vi "M02 Toy Factory.vi"(9 "Angle in":dbl format="%#_13g", 11 "EV3 in":T1) -> (3 "EV3 out":T1)   [LabVIEW 2016]
uses:
  <vilib>/NXT/Subs/LVHSConnector.ctl
  <vilib>/NXT/LegoClasses/BrickReference/BrickReference.lvclass
  <vilib>/NXT/Dual Mode Library/Waits/Wait_Num.vi
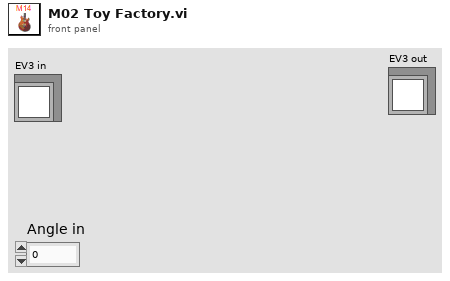
[diagram p1: front panel]
types:
  T1 = typedef "LVHSConnector.ctl" = refnum<class "BrickReference.lvclass">
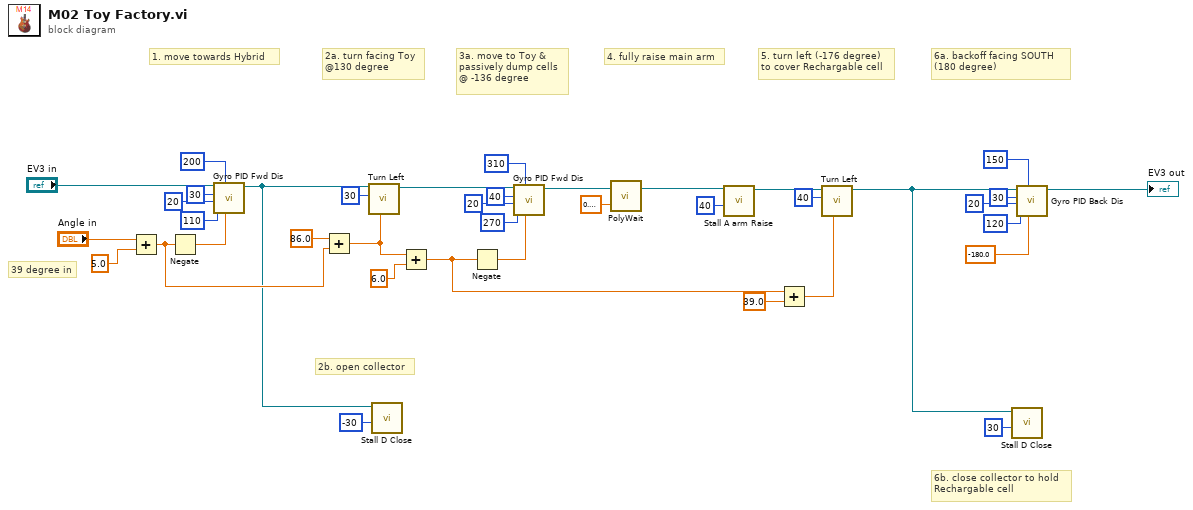
[diagram p0: block diagram]
diagram:
  # "39 degree in"
  # "6b. close collector to hold\nRechargable cell"
  # "2b. open collector"
  # "6a. backoff facing SOUTH\n(180 degree)"
  # "5. turn left (-176 degree)\nto cover Rechargable cell"
  # "4. fully raise main arm"
  # "3a. move to Toy &\npassively dump cells\n@ -136 degree"
  # "2a. turn facing Toy\n@130 degree"
  # "1. move towards Hybrid"
  n1 = Add(x="Angle in", y=5.0) -> (x+y=w30:dbl)
  n2 = Negate(x=w30) -> (-x=w28:dbl)
  n3 = call "Gyro PID Fwd Dis.vi"("Target angle"=w28, "Threshold to stop"=200 ("Stop rotation"), "Threshold to slow"=110 ("Threshold to De-acc"), "Min. speed"=20 ("De-acc"), "Max. speed"=30 ("Acc"), "EV3 in"="EV3 in") -> ("EV3 out"=w10:T1)  [unwired: 5 in]
  n4 = Add(x=86.0, y=w30) -> (x+y=w36:dbl)
  n5 = call "Turn Left.vi"("Turning angle"=w36, "Motor B (right)"=i8 30, "EV3 in"=w10) -> ("EV3 out"=w6:T1)  [unwired: 8 in]
  n6 = call "Stall D Close.vi"("Power"=i8 -30, "NXT/EV3"=w10) -> ()  [unwired: 9 in, 1 out]
  n7 = Add(x=w36, y=6.0) -> (x+y=w16:dbl)
  n8 = Negate(x=w16) -> (-x=w2:dbl)
  n9 = call "Gyro PID Fwd Dis.vi"("Target angle"=w2, "Threshold to stop"=310 ("Stop rotation"), "Threshold to slow"=270 ("Threshold to De-acc"), "Min. speed"=20 ("De-acc"), "Max. speed"=40 ("Acc"), "EV3 in"=w6) -> ("EV3 out"=w23:T1)  [unwired: 5 in]
  n10 = call-poly <vilib>:"PolyWait.vi"("Time (1 sec)"=sgl 0.7, "NXT/EV3"=w23) -> ("NXT/EV3"=w3:T1)  [unwired: 2 in]
  n11 = call "Stall A arm Raise.vi"("Power"=i8 40, "NXT/EV3"=w3) -> ("NXT/EV3"=w22:T1)  [unwired: 9 in]
  n12 = Add(x=w16, y=39.0) -> (x+y=w11:dbl)
  n13 = call "Turn Left.vi"("Turning angle"=w11, "Motor B (right)"=i8 40, "EV3 in"=w22) -> ("EV3 out"=w5:T1)  [unwired: 8 in]
  n14 = call "Stall D Close.vi"("Power"=i8 30, "NXT/EV3"=w5) -> ()  [unwired: 9 in, 1 out]
  n15 = call "Gyro PID Back Dis.vi"("Target angle"=sgl -180.0, "Threshold to stop"=150, "Threshold to slow"=120, "Min. speed"=20, "Max. speed"=30, "EV3 in"=w5) -> ("EV3 out"=→"EV3 out":T1)  [unwired: 5 in]
